vi "GetTorqueRipple.vi"(5 "3-phases voltage waveforms":waveform(dbl)[](array[waveform]), 6 "Calculation State in":T3, 7 "3-phase current waveforms":waveform(dbl)[](array[waveform]), 8 "error in (no error)":errorcluster, 9 "Motor info":T1, 10 "Channel":T6, 11 "data map":T2) -> (0 "error out":errorcluster, 1 "invalid estimation":bool, 2 "Torque Ripple (%)":dbl, 3 "data map out":T2, 4 "Calculation State out":T3)   [LabVIEW 2017, in "McsaAnalysisFunctions.lvlib"]
uses:
  <vilib>/addons/InsightCM/Utilities/Analysis/MCSA/McsaAnalysisFunctions.lvlib
  <vilib>/addons/PointValueMap/controls/PointMap.ctl
  <vilib>/addons/InsightCM/Utilities/Analysis/MCSA/controls/McsaChannel.ctl
  <vilib>/addons/InsightCM/Utilities/Analysis/Shared/controls/Feature.ctl
  <vilib>/addons/InsightCM/Utilities/Analysis/Shared/controls/AmplitudeScale.ctl
  <vilib>/addons/InsightCM/MessageBus/Base/controls/KeyValuePair.ctl
  <vilib>/addons/InsightCM/Utilities/Analysis/MCSA/controls/MotorCalculationCache.ctl
  <vilib>/addons/Electrical Power/Basic/Measurement/subVIs/basic_Power Value.ctl
  <vilib>/addons/InsightCM/Utilities/Analysis/MCSA/controls/TorqueLoadEfficiency.ctl
  <vilib>/addons/InsightCM/Utilities/Analysis/MCSA/controls/McsaMotor.ctl
  <vilib>/addons/Electrical Power/Motor Monitoring/Torque, Load, and Efficiency (Air Gap, N Motors).vi
  <vilib>/addons/Electrical Power/Motor Monitoring/NI_EP_Motor Monitoring.lvlib
  <vilib>/addons/PointValueMap/PointValueMap.lvlib
  <vilib>/addons/InsightCM/Utilities/Analysis/Shared/AnalysisHelper.lvlib
  <vilib>/addons/Electrical Power/Basic/NI_EP_Basic.lvlib
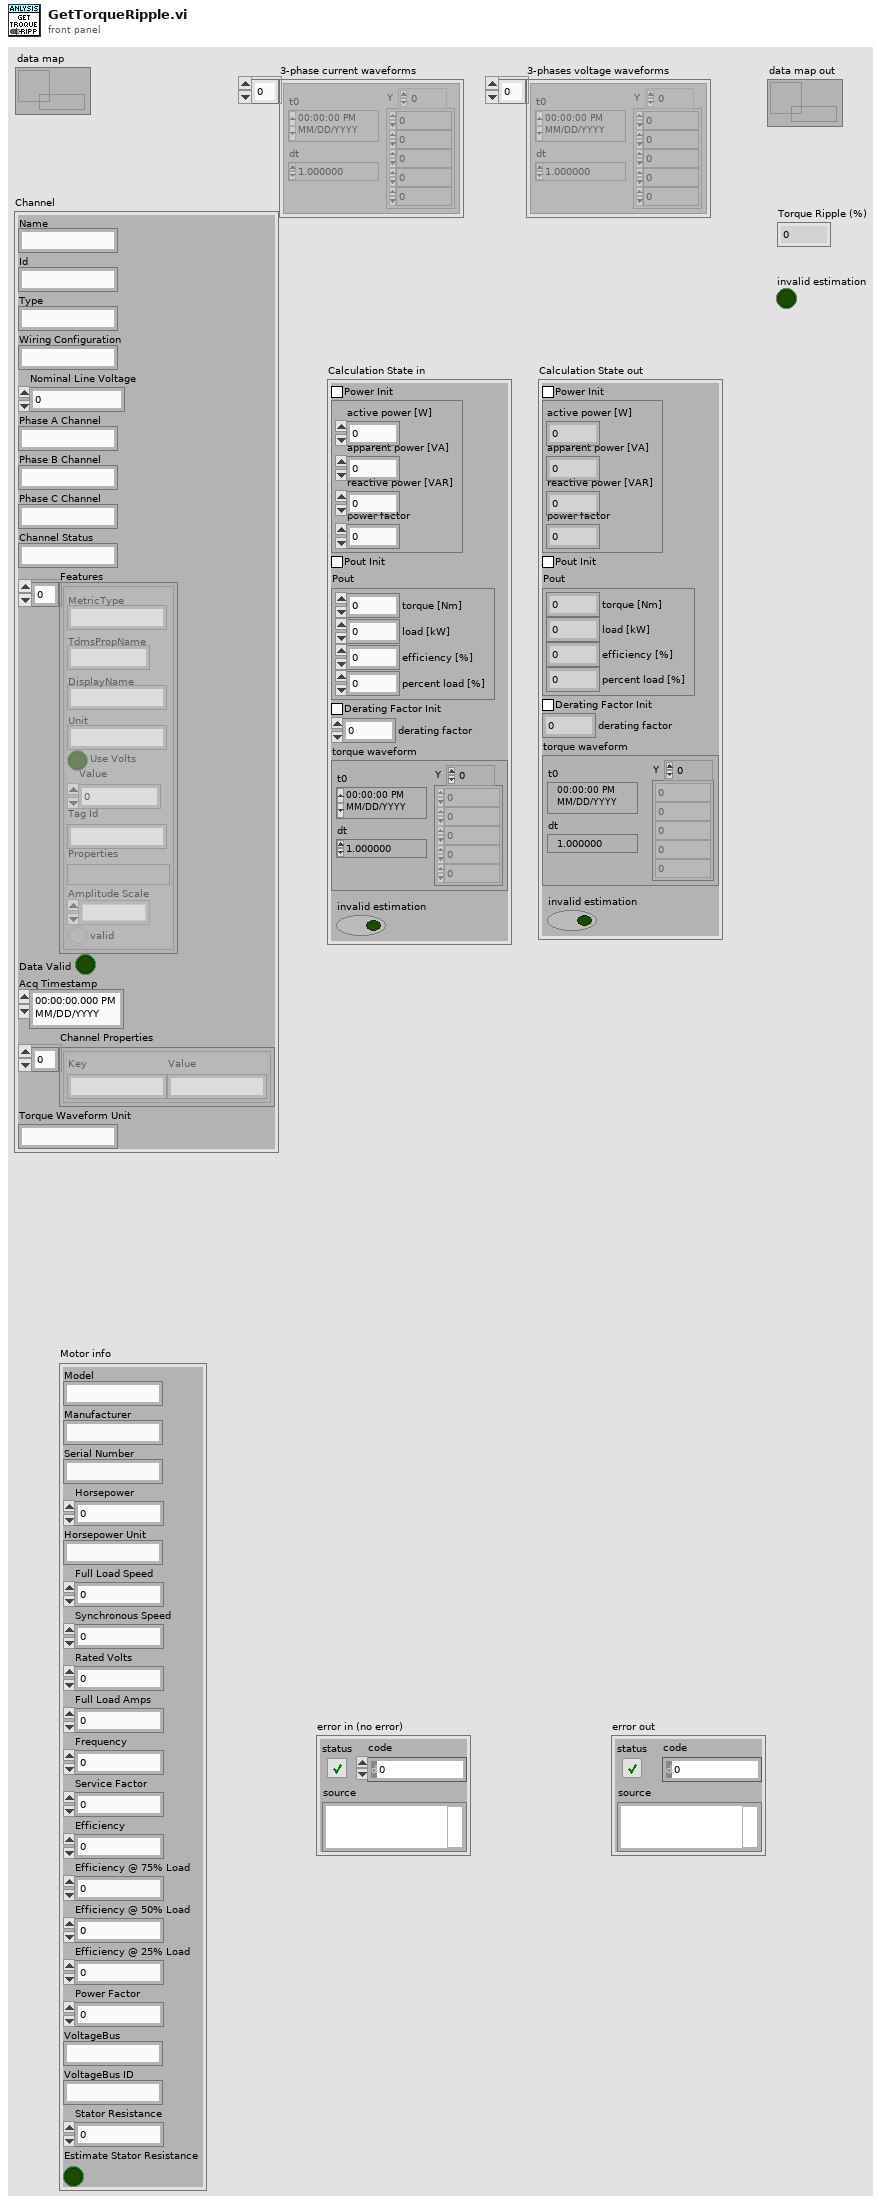
[diagram p1: front panel]
types:
  T1 = typedef "McsaAnalysisFunctions.lvlib/McsaMotor.ctl" = cluster{"Model":string, "Manufacturer":string, "Serial Number":string, "Horsepower":dbl, "Horsepower Unit":string, "Full Load Speed":dbl, "Synchronous Speed":dbl, "Rated Volts":dbl, "Full Load Amps":dbl, "Frequency":dbl, "Service Factor":dbl, "Efficiency":dbl, "Efficiency @ 75% Load":dbl, "Efficiency @ 50% Load":dbl, "Efficiency @ 25% Load":dbl, "Power Factor":dbl, "VoltageBus":string, "VoltageBus ID":string, "Stator Resistance":dbl, "Estimate Stator Resistance":bool}
  T2 = typedef "PointValueMap.lvlib/PointMap.ctl" = refnum<data-value>
  T3 = typedef "McsaAnalysisFunctions.lvlib/MotorCalculationCache.ctl" = cluster{"Power Init":bool, "power value":T4, "Pout Init":bool, "Pout":T5, "Derating Factor Init":bool, "derating factor":sgl, "torque waveform":waveform(dbl), "invalid estimation":bool}
  T4 = typedef "NI_EP_Basic.lvlib/basic_Power Value.ctl" = cluster{"active power [W]":dbl, "apparent power [VA]":dbl, "reactive power [VAR]":dbl, "power factor":dbl}
  T5 = typedef "McsaAnalysisFunctions.lvlib/TorqueLoadEfficiency.ctl" = cluster{"torque [Nm]":dbl, "load [kW]":dbl, "efficiency [%]":dbl, "percent load [%]":dbl}
  T6 = typedef "McsaAnalysisFunctions.lvlib/McsaChannel.ctl" = cluster{"Name":string, "Id":string, "Type":string, "Wiring Configuration":string, "Nominal Line Voltage":dbl, "Phase A Channel":string, "Phase B Channel":string, "Phase C Channel":string, "Channel Status":string, "Features":T7[], "Data Valid":bool, "Acq Timestamp":timestamp, "Channel Properties":T9[], "Torque Waveform Unit":string}
  T7 = typedef "AnalysisHelper.lvlib/Feature.ctl" = cluster{"MetricType":string, "TdmsPropName":string, "DisplayName":string, "Unit":string, "Use Volts":bool, "Value":dbl, "Tag Id":string, "Properties":variant, "Amplitude Scale":T8, "valid":bool}
  T8 = typedef "AnalysisHelper.lvlib/AmplitudeScale.ctl" = enum16{"rms", "peak", "pk-pk"}
  T9 = typedef "KeyValuePair.ctl" = cluster{"Key":string, "Value":string}
  T10 = cluster{"nominal frequency":enum16{"50 Hz", "60 Hz"}, "motor information":cluster{"synchronous speed [RPM]":dbl, "full load [kW]":dbl, "full load efficiency [%]":dbl}[]}
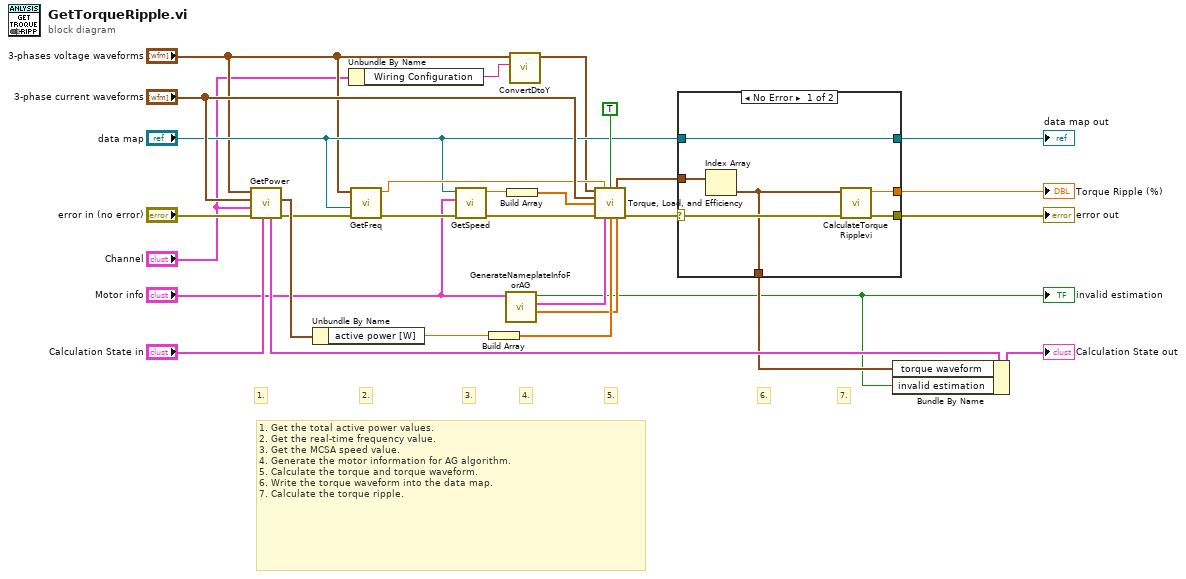
[diagram p0: block diagram]
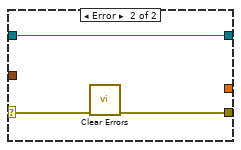
[diagram p2: hidden frame]
diagram:
  # "7."
  # "1. Get the total active power values.\n2. Get the real-time frequency value.\n3. Get the MCSA speed value.\n4. Generate the motor information for AG algorithm.\n5. Calculate the torque and torque waveform.\n6. Write the torque waveform into the data map.\n7. Calculate the torque ripple."
  # "6."
  # "5."
  # "4."
  # "3."
  # "2."
  # "1."
  n1 = call <vilib>:"GetPower.vi"("Calculation State in"="Calculation State in", "error in (no error)"="error in (no error)", "Channel"="Channel", "3-phase current waveform"="3-phase current waveforms", "3-phase voltage waveform"="3-phases voltage waveforms") -> ("error out"=w26:errorcluster, "power value"=w29:T4, "Calculation State out"=w28:T3)  [unwired: 4 in]
  n2 = Unbundle By Name(w29) -> ("active power [W]"=w20:dbl)
  n3 = Unbundle By Name("Channel") -> ("Wiring Configuration"=w5:string)
  n4 = call <vilib>:"GetFreq.vi"("error in (no error)"=w26, "Map"="data map", "waveforms"="3-phases voltage waveforms") -> ("error out"=w25:errorcluster, "frequency"=w23:dbl)  [unwired: 7 in]
  n5 = call <vilib>:"GetSpeed.vi"("error in (no error)"=w25, "Motor"="Motor info", "Map"="data map") -> ("error out"=w11:errorcluster, "Speed [RPM]"=w22:dbl)  [unwired: 7 in]
  n6 = Build Array(w20) -> (w19:dbl[])
  n7 = call <vilib>:"GenerateNameplateInfoForAG.vi"("motor nameplate information"="Motor info") -> ("stator resistance"=w18:dbl[], "nameplate information for AG"=w14:T10, "invalid stator resistance"=w1:bool)  [unwired: 8 in]
  "invalid estimation" <- w1
  n8 = Build Array(w22) -> (w21:dbl[])
  n9 = call <vilib>:"ConvertDtoY.vi"("Wiring Configuration"=w5, "voltage waveform"="3-phases voltage waveforms") -> ("phase voltage waveform"=w8:waveform(dbl)[])  [unwired: 8 in, 1 out]
  n10 = call-poly <vilib>:"Torque, Load, and Efficiency.vi"("phase voltage waveforms"=w8, "fundamental frequency [Hz]"=w23, "reset? (F)"=TRUE, "current waveforms"="3-phase current waveforms", "speed [RPM]"=w21, "error in (no error)"=w11, "nameplate information"=w14, "total input active power [W]"=w19, "stator resistance [ohms]"=w18) -> ("torque waveforms [Nm]"=w17:waveform(dbl)[], "error out"=w10:errorcluster)  [unwired: 2 in, 3 out]
  n11 = case shown="No Error" w10 {
    selector: w10 -> [w32 w39]
    tunnel: w17 -> [w36 _]
    tunnel: [w35 w38] -> w16
    tunnel: [w34 _] -> w2
    tunnel: "data map" -> [w33 w37]
    tunnel: [w33 w37] -> w9
    tunnel: [w31 _] -> w3
    frame No Error {
      n12 = Index Array(array=w36) -> (element=w31:waveform(dbl))  [unwired: 1 in]
      n13 = call <vilib>:"CalculateTorqueRipplevi.vi"("error in (no error)"=w32, "Torque Waveform"=w31) -> ("error out"=w35:errorcluster, "Torque Ripple (%)"=w34:dbl)  [unwired: 8 in]
    }
    frame Error {
      n14 = call <vilib>:"Clear Errors.vi"("error in (no error)"=w39) -> ("error out"=w38:errorcluster)  [unwired: 5 in, 1 out]
    }
  }
  "Torque Ripple (%)" <- w2
  "error out" <- w16
  "data map out" <- w9
  n15 = Bundle By Name(cluster=w28, "torque waveform"=w3, "invalid estimation"=w1) -> (→"Calculation State out":T3)
